vi "Merge Game and Move Views.vi"(7 "Team Index":i32, 10 "Move View Out":i32[](array[numeric]), 11 "System View Out":i32[](array[numeric])) -> (3 "New View Out":i32[](array[numeric]))   [LabVIEW 2017, in "AntFarm_MB.lvclass"]
uses:
  AntFarm_MB.lvclass
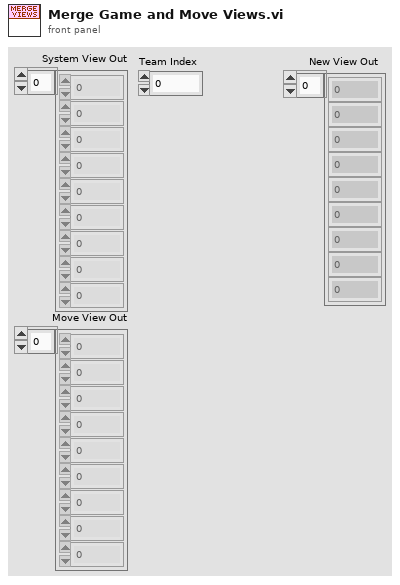
[diagram p1: front panel]
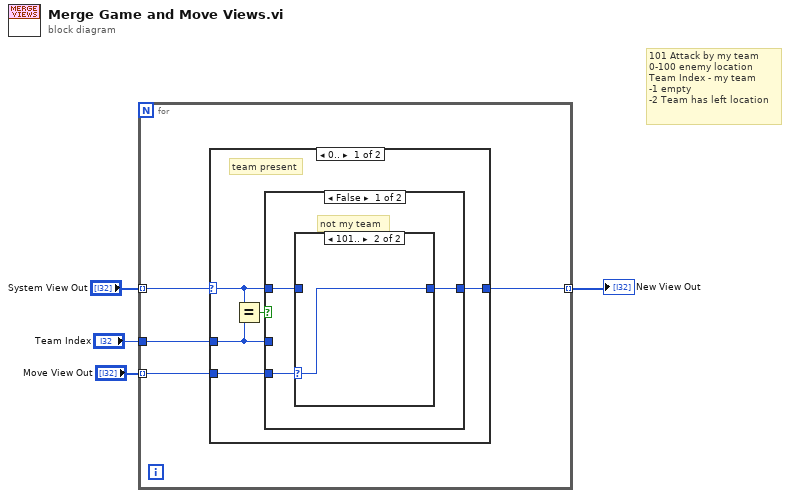
[diagram p0: block diagram]
diagram:
  # "101 Attack by my team\n0-100 enemy location\nTeam Index - my team\n-1 empty\n-2 Team has left location"
  n1 = for {
    tunnel: "System View Out" -> [w8] mode=indexing
    tunnel: "Move View Out" -> [w6] mode=indexing
    tunnel: "Team Index" -> [w5]
    tunnel: [w7] -> w1 mode=indexing
    n2 = case shown="0.." w8 {
      selector: w8 -> [w12 _]
      tunnel: [w10 w24] -> w7
      tunnel: w6 -> [w11 w24]
      tunnel: w5 -> [w9 _]
      frame 0.. {
        # "team present"
        n3 = Equal?(x=w12, y=w9) -> (x = y?=w13:bool)
        n4 = case shown="False" w13 {
          tunnel: w12 -> [w14 w19]
          tunnel: w11 -> [w16 w21]
          tunnel: [w15 w20] -> w10
          tunnel: w9 -> [_ _]
          frame False {
            # "not my team"
            n5 = case shown="101.." w16 {
              selector: w16 -> [_ w18]
              tunnel: [w17 w18] -> w15
              tunnel: w14 -> [w17 _]
              frame ..100 {
              }
              frame 101.. {
              }
            }
          }
          frame True {
            # "my team"
            n6 = case shown="..-2" w21 {
              selector: w21 -> [_ w23]
              tunnel: [w22 w23] -> w20
              tunnel: w19 -> [w22 _]
              frame -1.. {
              }
              frame ..-2 {
                # "Teammate move\noff location"
              }
            }
          }
        }
      }
      frame ..-1 {
        # "Move team Present"
        # "System empty"
      }
    }
  }
  "New View Out" <- w1
